vi "F020_sn_set.vi"(8 "error in":errorcluster, 10 "Cluster":cluster{"address":u32, "SN":u32} {"SN" format="%08x"; "address" format="%02x"}, 11 "COM in":string="}") -> (0 "error out":errorcluster, 3 "COM out":string="}")   [LabVIEW 2016]
doc: "This example performs a serial port write and a serial port read. The parameters set for the serial port must match the parameters of the connected instrument or device. The VISA Configure Serial Port VI sets the configuration parameters. The front panel displays the controls used to configure the basic parameters, such as baud rate, data bits, and parity. The VI passes the VISA resource name to other VIs that perform operations on that VISA resource. The VISA Write function sends a command to the serial device and the VISA Read function returns data based on the command. The VISA Close function then closes the reference to the serial device. It is important to close the reference; otherwise, further communication through that port might not be possible."
panel:
  # "loopback: <xxAABB>\nwr_dout:   <xxAA11aabbccdd> aa=ch, bb=val, ccdd=timeout[sec]"
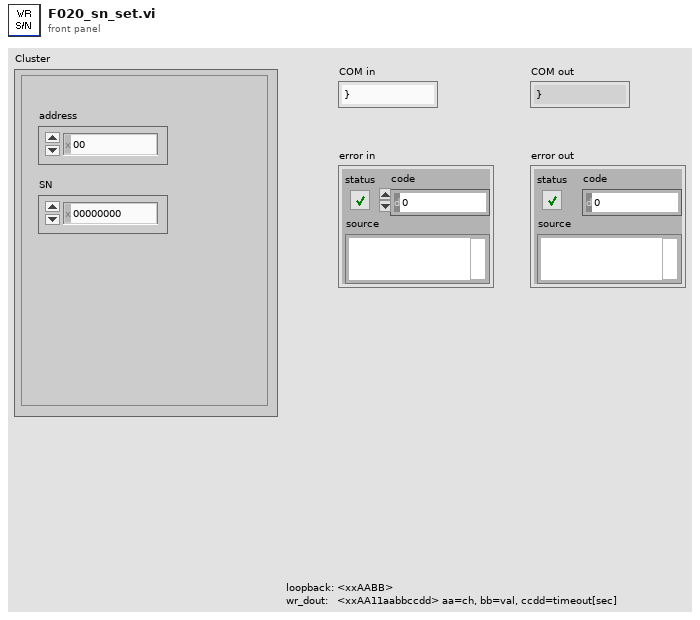
[diagram p1: front panel]
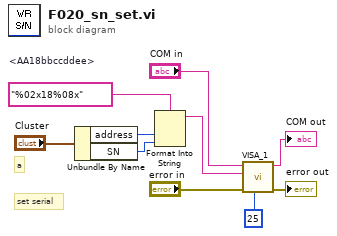
[diagram p0: block diagram]
diagram:
  w7 = "%02x18%08x"  # <AA18bbccddee>
  # "set serial"
  # "a"
  n1 = Unbundle By Name("Cluster") -> ("address"=w4:u32, "SN"=w5:u32)
  n2 = Format Into String(format string=w7, w4, w5) -> (resulting string=w1:string)  [unwired: 2 in, 1 out]
  n3 = call "VISA_1.vi"("delay[ms]"=u32 25, "error in"="error in", "wr_buf"=w1, "COM in"="COM in") -> ("error out"=→"error out":errorcluster, "COM out"=→"COM out":string)  [unwired: 4 in, 2 out]
